vi "From Variant.vi"(8 "error in (no error)":errorcluster, 10 "Variant":variant, 11 "Abs_Waveform in":refnum<class "Abs_Waveform.lvclass">) -> (0 "error out":errorcluster, 3 "Abs_Waveform out":refnum<class "Abs_Waveform.lvclass">)   [LabVIEW 2021, in "Abs_Waveform.lvclass"]
uses:
  Abs_Waveform.lvclass
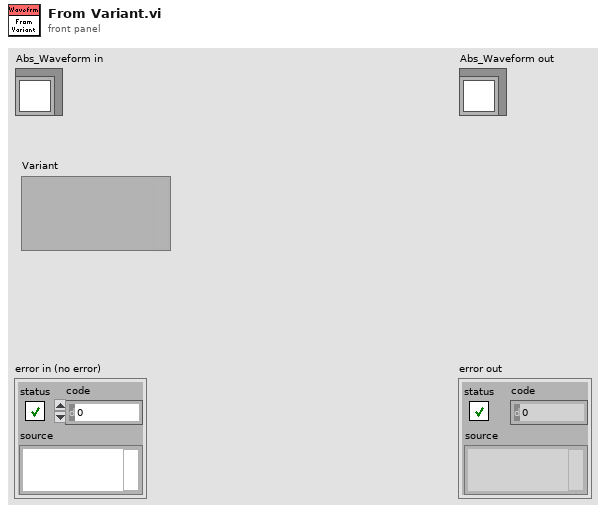
[diagram p1: front panel]
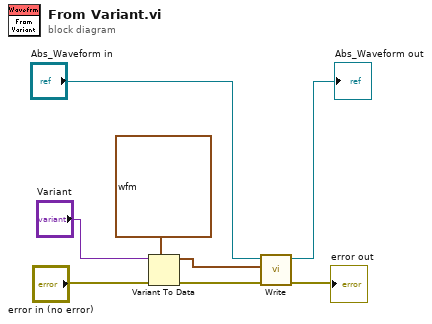
[diagram p0: block diagram]
diagram:
  n1 = Variant To Data(error in="error in (no error)", type=waveform(dbl) {"t0"=timestamp(0 s since 1904-01-01), "dt"=1.0, "Y"=[]}, Variant="Variant") -> (data=w5:waveform(dbl), error out=w6:errorcluster)
  n2 = call-dynamic "Write.vi"("error in (no error)"=w6, "Waveform"=w5, "Abs_Waveform in"="Abs_Waveform in") -> ("error out"=→"error out":errorcluster, "Abs_Waveform out"=→"Abs_Waveform out":refnum<class "Abs_Waveform.lvclass">)  [unwired: 7 in]
